vi "WPI_AnalogChannelGetAverageVoltageNavX.vi"(8 "error in":errorcluster, 11 "AIDeviceRef":T1={"DevStatus"={"status"=FALSE, "code"=0, "source"=""}, "Analog Channel"=enum."AI 1"}) -> (0 "error out":errorcluster, 2 "Voltage":dbl, 3 "AIDeviceRef":T1={"DevStatus"={"status"=FALSE, "code"=0, "source"=""}, "Analog Channel"=enum."AI 1"})   [LabVIEW 2016]
doc: "Returns the average voltage value from the oversample and average engine for the channel. The converter scales the raw value to the voltage value using the least significant bit weight constant and the offset constant of the hardware. Oversampling increases the resolution of the voltage value but decreases the update rate. Averaging returns a stable voltage value but also decreases the update rate. Use the GetVoltage VI to get voltage values directly from the A/D converter.\n\nThis software is licensed. Open the labview\\readme\\WPI Robotics Library Open Source License.txt file for more information."
uses:
  <vilib>/Rock Robotics/WPI/AnalogChannel/WPI_AnalogChannelDevRef.ctl
  <vilib>/Rock Robotics/SystemInterfaces/AI/FPGA_AIChannel.ctl
  <vilib>/ptbypt/NI_PtbyPt.lvlib
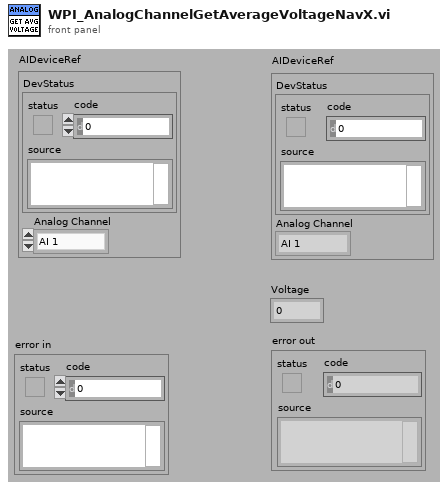
[diagram p1: front panel]
types:
  T1 = typedef "WPI_AnalogChannelDevRef.ctl" = cluster{"DevStatus":errorcluster, "Analog Channel":T2}
  T2 = typedef "FPGA_AIChannel.ctl" = enum8{"AI 0", "AI 1", "AI 2", "AI 3", "AI MXP 0", "AI MXP 1", "AI MXP 2", "AI MXP 3", "Invalid"}
  T3 = typedef "WPI_AnalogModuleDevStatus.ctl" = cluster{"DevStatus":errorcluster}
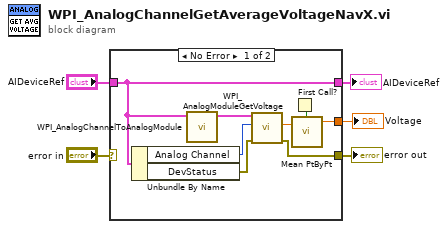
[diagram p0: block diagram]
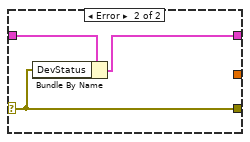
[diagram p2: hidden frame]
diagram:
  n1 = case shown="No Error" "error in" {
    selector: "error in" -> [_ w14]
    tunnel: "AIDeviceRef" -> [w13 w16]
    tunnel: [w13 w15] -> w4
    tunnel: [w8 _] -> w3
    tunnel: [w9 w14] -> w1
    frame No Error {
      n2 = Unbundle By Name(w13) -> ("Analog Channel"=w12:T2, "DevStatus"=w10:errorcluster)
      n3 = call <vilib>:"WPI_AnalogChannelToAnalogModule.vi"("AIDeviceRef"=w13) -> ("AIDeviceRef"=w11:T3)  [unwired: 10 out]
      n4 = call <vilib>:"WPI_AnalogModuleGetVoltage.vi"("error in (no error)"=w10, "Channel"=w12, "AnalogModuleDevRef"=w11) -> ("error out"=w9:errorcluster, "Voltage"=w7:dbl)  [unwired: 6 in, 1 out]
      n5 = First Call?() -> (First Call?: T/F=w6:bool)
      n6 = call <vilib>:"Mean PtByPt.vi"("x"=w7, "initialize"=w6) -> ("mean"=w8:dbl)  [unwired: 2 in, 1 out]
    }
    frame Error {
      n7 = Bundle By Name(cluster=w16, "DevStatus"=w14) -> (w15:T1)
    }
  }
  "AIDeviceRef" <- w4
  "Voltage" <- w3
  "error out" <- w1
